vi "Actor Core.vi"(8 "error in":errorcluster, 11 "Generator Base in":refnum<class "Generator Base.lvclass">) -> (0 "error out":errorcluster, 3 "Actor out":refnum<class "Actor.lvclass">)   [LabVIEW 2018, in "Generator Base.lvlib" / "Generator Base.lvclass"]
doc: "(<B>Filename</B>: Actor Framework.lvlib:Actor.lvclass:Actor Core.vi)\n\nReceives messages to the actor, reacts to them, and initiates any error handling that may shut the actor down.\n\nDescendant classes may override this VI to append parallel tasks for the actor to complete while it handles messages. Overrides use the Call Parent Method node."
uses:
  Generator Base.lvclass
  <vilib>/ActorFramework/Actor/Actor.lvclass
  Generator Base Messages/Update Msg/Update Msg.lvclass
  <vilib>/NI/Event Source Actor/Event Source/Event Source/Event Source.lvclass
  C:/Program Files (x86)/National Instruments/LabVIEW 2018/vi.lib/NI/Event Source Actor/Event Source/Event Source/Event Source.lvclass
  C:/Program Files (x86)/National Instruments/LabVIEW 2018/vi.lib/ActorFramework/Actor/Actor.lvclass
  C:/Program Files (x86)/National Instruments/LabVIEW 2018/vi.lib/ActorFramework/Message/Message.lvclass
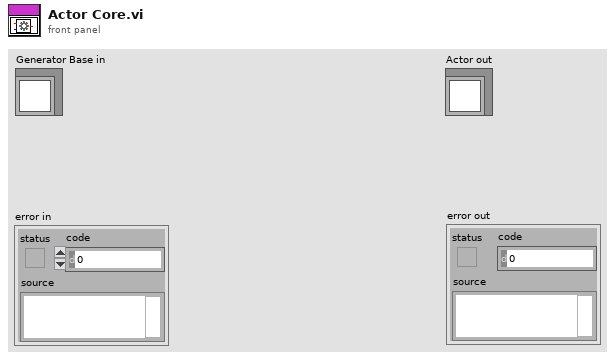
[diagram p1: front panel]
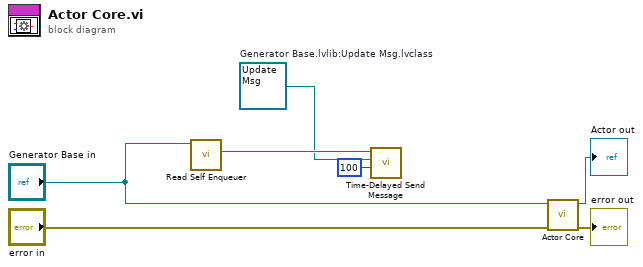
[diagram p0: block diagram]
diagram:
  w2 = refnum<class "Update Msg.lvclass"> refnum  # Generator Base.lvlib:Update Msg.lvclass
  n1 = call <vilib>:"Read Self Enqueuer.vi"("Actor"="Generator Base in") -> ("Self Enqueuer"=w3:refnum<class "Message Enqueuer.lvclass">)  [unwired: 10 in]
  n2 = call <vilib>:"Time-Delayed Send Message.vi"("Milliseconds To Wait"=100, "Message"=w2, "Message Enqueuer"=w3) -> ()  [unwired: 7 in, 2 out]
  n3 = call-parent "Actor Core.vi"("error in"="error in", "Actor in"="Generator Base in") -> ("error out"=→"error out":errorcluster, "Actor out"=→"Actor out":refnum<class "Actor.lvclass">)  [unwired: 8 in]
